vi "Build Private Data.vi"(8 "error in (no error)":errorcluster, 10 "Wiring Spec":T1, 11 "CS++Actor in":refnum<class "CS++Actor.lvclass">) -> (0 "error out":errorcluster, 3 "CS++Actor out":refnum<class "CS++Actor.lvclass">)   [LabVIEW 2014, in "CS++Actor.lvlib" / "CS++Actor.lvclass"]
doc: "creates the attribute data of the new message."
uses:
  CS++Actor.lvclass
  <vilib>/Utility/traverseref.llb/TRef TravTarget.ctl
  CS++Actor.lvclass/CS++Actor.ctl
  <vilib>/Utility/miscctls.llb/LVPositionTypeDef.ctl
  <vilib>/Utility/traverseref.llb/VI Scripting - Traverse.lvlib
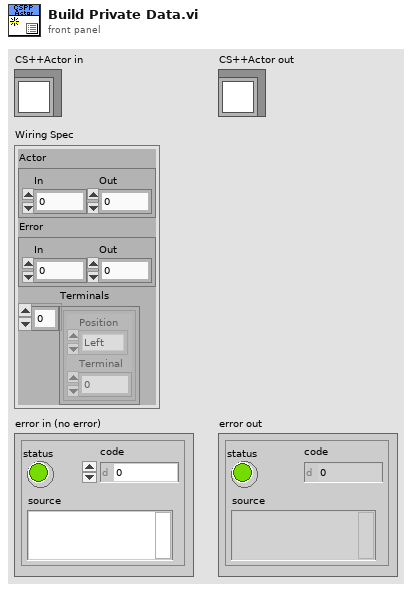
[diagram p1: front panel]
types:
  T1 = cluster{"Actor":cluster{"In":i32, "Out":i32}, "Error":cluster{"In":i32, "Out":i32}, "Terminals":cluster{"Position":enum16{"Left", "Top", "Bottom", "Right"}, "Terminal":i32}[]}
  T2 = typedef "TRef TravTarget.ctl" = enum16{"FP", "BD", "Other"}
  T3 = typedef "LVPositionTypeDef.ctl" = cluster{"Left":i32, "Top":i32}
  T4 = cluster{"Position":enum16{"Left", "Top", "Bottom", "Right"}, "Terminal":i32}[]
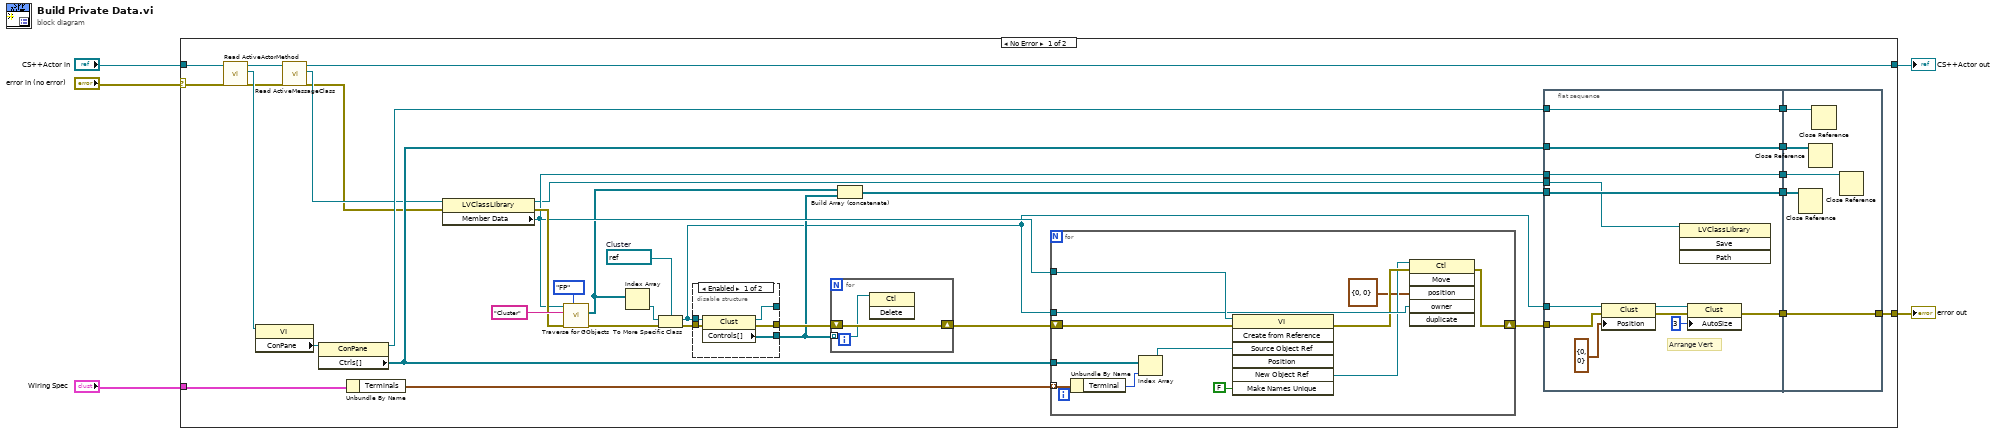
[diagram p0: block diagram]
diagram:
  n1 = case shown="No Error" "error in (no error)" {
    selector: "error in (no error)" -> [w7 w80]
    tunnel: [w26 w80] -> w5
    tunnel: "Wiring Spec" -> [w24 _]
    tunnel: "CS++Actor in" -> [w13 w79]
    tunnel: [w10 w79] -> w2
    frame No Error {
      w30 = refnum<vi> refnum  # Cluster
      n2 = call "Read ActiveActorMethod.vi"("error in (no error)"=w7, "CS++Actor in"=w13) -> ("error out"=w9:errorcluster, "ActiveActorMethod"=w11:refnum<vi>, "CS++Actor out"=w12:refnum<class "CS++Actor.lvclass">)  [unwired: 7 in]
      n3 = property class="VI"(reference=w11) -> ("ConPane"=w35:refnum<vi>)  [unwired: 1 in, 2 out]
      n4 = call "Read ActiveMessageClass.vi"("error in (no error)"=w9, "CS++Actor in"=w12) -> ("error out"=w8:errorcluster, "ActiveMessageClass"=w14:refnum<vi>, "CS++Actor out"=w10:refnum<class "CS++Actor.lvclass">)  [unwired: 7 in]
      n5 = property class="ConPane"(reference=w35) -> (reference out=w16:refnum<vi>, "Ctrls[]"=w25:refnum<vi>[])  [unwired: 1 in, 1 out]
      n6 = Unbundle By Name(w24) -> ("Terminals"=w23:T4)
      n7 = property class="LVClassLibrary"(reference=w14, error in=w8) -> (reference out=w15:refnum<vi>, error out=w32:errorcluster, "Member Data"=w28:refnum<vi>)
      n8 = call <vilib>:"Traverse for GObjects.vi"("Traverse Target"=TRef_TravTarget."FP", "error in (no error)"=w32, "Class Name"="Cluster" ("name/order"), "VI Refnum"=w28) -> ("error out"=w29:errorcluster, "References"=w27:refnum<vi>[])  [unwired: 4 in, 2 out]
      n9 = Index Array(array=w27) -> (element=w31:refnum<vi>)  [unwired: 1 in]
      n10 = To More Specific Class(target class=w30, reference=w31, error in=w29) -> (specific class reference=w6:refnum<vi>, error out=w22:errorcluster)
      n11 = disable-structure shown="Enabled" {
        disable-tunnel: w6 -> [w47 w49]
        disable-tunnel: w22 -> [w46 w48]
        disable-tunnel: [w45 w49] -> _
        disable-tunnel: [w44 w48] -> w20
        disable-tunnel: [w43 _] -> w17
        frame Enabled {
          n12 = property class="Clust"(reference=w47, error in=w46) -> (reference out=w45:refnum<vi>, error out=w44:errorcluster, "Controls[]"=w43:refnum<vi>[])
        }
        frame Disabled {
        }
      }
      n13 = for {
        shift-right: [w42] -> w19
        shift-left: w20 -> [w42]
        tunnel: w17 -> [w41] mode=indexing
        n14 = invoke class="Ctl" method="Delete"(reference=w41) -> ()  [unwired: 2 in, 3 out]
      }
      n15 = Build Array (concatenate)(w27, w17) -> (w18:refnum<vi>[])
      n16 = for {
        tunnel: w25 -> [w74]
        tunnel: w28 -> [w78]
        shift-right: [w77] -> w21
        shift-left: w19 -> [w72]
        tunnel: w23 -> [w73] mode=indexing
        tunnel: w6 -> [w76]
        n17 = Unbundle By Name(w73) -> ("Terminal"=w71:i32)
        n18 = Index Array(array=w74, index=w71) -> (element=w70:refnum<vi>)
        n19 = invoke class="VI" method="Create from Reference"(reference=w78, error in=w72, "Source Object Ref"=w70, "Make Names Unique"=FALSE ("Make Names Unique (F)")) -> (error out=w75:errorcluster, "New Object Ref"=w69:refnum<vi>)  [unwired: 3 in, 5 out]
        n20 = invoke class="Ctl" method="Move"(reference=w69, error in=w75, "position"=T3 {"Left"=0, "Top"=0}, "owner"=w76) -> (error out=w77:errorcluster)  [unwired: 2 in, 5 out]
      }
      n21 = flat-sequence {
        tunnel: w6 -> [w61]
        tunnel: w21 -> [w56]
        tunnel: w28 -> [w53]
        tunnel: w18 -> [w55]
        tunnel: [w52] -> w40
        tunnel: [w53] -> w39
        tunnel: [w55] -> w38
        tunnel: w25 -> [w54]
        tunnel: [w54] -> w37
        tunnel: w16 -> [w51]
        tunnel: [w51] -> w36
        tunnel: w15 -> [w50]
        tunnel: [w66] -> w26
        tunnel: w40 -> [w66]
        tunnel: w39 -> [w65]
        tunnel: w38 -> [w64]
        tunnel: w37 -> [w63]
        tunnel: w36 -> [w62]
        frame #0 {
          # "Arrange Vert"
          n22 = property class="Clust"(reference=w61, error in=w56, "Position"=T3 {"Left"=0, "Top"=0}) -> (reference out=w59:refnum<vi>, error out=w58:errorcluster)
          n23 = invoke class="LVClassLibrary" method="Save"(reference=w50) -> ()  [unwired: 3 in, 4 out]
          n24 = property class="Clust"(reference=w59, error in=w58, "AutoSize"=u32 3 ("Auto Sizing")) -> (error out=w52:errorcluster)  [unwired: 1 out]
        }
        frame #1 {
          n25 = Close Reference(reference=w64) -> ()  [unwired: 1 in, 1 out]
          n26 = Close Reference(reference=w63) -> ()  [unwired: 1 in, 1 out]
          n27 = Close Reference(reference=w62) -> ()  [unwired: 1 in, 1 out]
          n28 = Close Reference(reference=w65) -> ()  [unwired: 1 in, 1 out]
        }
      }
    }
    frame Error {
    }
  }
  "error out" <- w5
  "CS++Actor out" <- w2
